vi "PID Resize 1D Cluster Array.vi"(4 "array size":i32, 5 "input array":cluster{"output high":dbl, "output low":dbl}[](array[cluster]) {"output low" format="%.2f"; "output high" format="%.2f"}) -> (2 "output array":cluster{"output high":dbl, "output low":dbl}[](array[cluster]) {"output low" format="%.2f"; "output high" format="%.2f"})   [LabVIEW 2017, in "NI_PID_pid.lvlib"]
uses:
  <vilib>/addons/control/pid/NI_PID_pid.lvlib
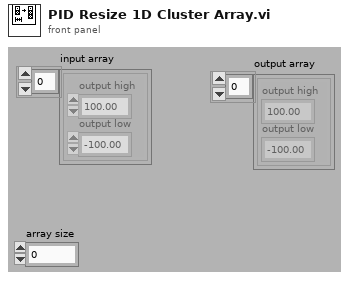
[diagram p1: front panel]
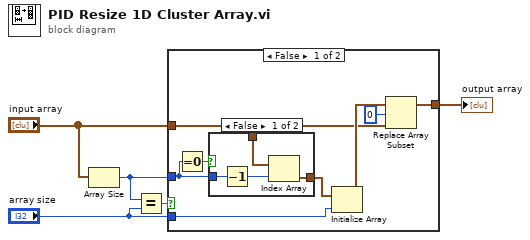
[diagram p0: block diagram]
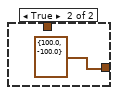
[diagram p2: hidden frame]
diagram:
  n1 = Array Size(array="input array") -> (size(s)=w4:i32)
  n2 = Equal?(x=w4, y="array size") -> (x = y?=w5:bool)
  n3 = case shown="False" w5 {
    tunnel: "input array" -> [w9 w19]
    tunnel: [w13 w19] -> w1
    tunnel: "array size" -> [w12 _]
    tunnel: w4 -> [w7 _]
    frame False {
      n4 = Equal To 0?(x=w7) -> (x = 0?=w6:bool)
      n5 = case shown="False" w6 {
        tunnel: w7 -> [w17 _]
        tunnel: [w15 cluster{"output high":dbl, "output low":dbl} {"output high"=100.0, "output low"=-100.0} ("output range 2")] -> w11
        tunnel: w9 -> [w14 _]
        frame False {
          n6 = Decrement(x=w17) -> (x-1=w16:i32)
          n7 = Index Array(array=w14, index=w16) -> (element=w15:cluster{"output high":dbl, "output low":dbl})
        }
        frame True {
        }
      }
      n8 = Initialize Array(w11, w12) -> (w10:cluster{"output high":dbl, "output low":dbl}[])
      n9 = Replace Array Subset(array=w10, new element=w9, index=0) -> (w13:cluster{"output high":dbl, "output low":dbl}[])
    }
    frame True {
    }
  }
  "output array" <- w1
